vi "TCP Client_Get data signals.vi"(6 "error in":errorcluster, 7 "timeout ms":i32, 8 "hostname":string, 9 "Port":i32) -> (0 "error out":errorcluster, 1 "Array2D":sgl[][](array[numeric]), 2 "Array":sgl[](array[numeric]), 3 "Signals_names":string[](array[string]))   [LabVIEW 2022 SP3]
panel:
  out "R_message 1":string
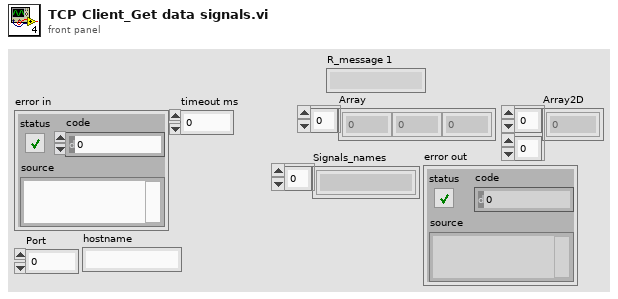
[diagram p1: front panel]
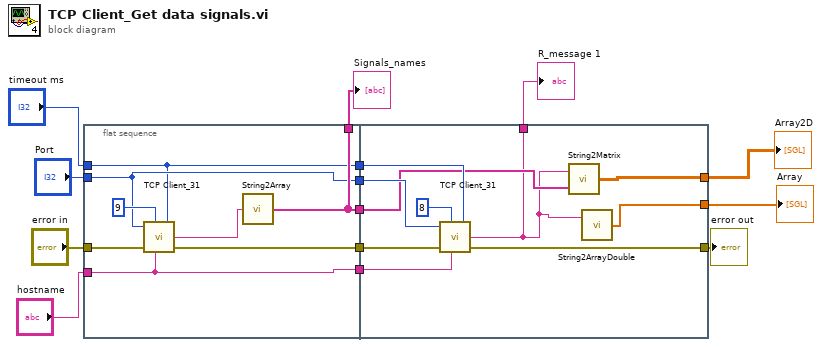
[diagram p0: block diagram]
diagram:
  n1 = flat-sequence {
    tunnel: [w18] -> w14
    tunnel: "error in" -> [w20]
    tunnel: [w19] -> w13
    tunnel: [w18] -> w5
    tunnel: "Port" -> [w17]
    tunnel: [w17] -> w10
    tunnel: "hostname" -> [w16]
    tunnel: [w16] -> w8
    tunnel: "timeout ms" -> [w15]
    tunnel: [w15] -> w6
    tunnel: w14 -> [w25]
    tunnel: w13 -> [w32]
    tunnel: [w31] -> w4
    tunnel: w10 -> [w29]
    tunnel: w8 -> [w28]
    tunnel: w6 -> [w27]
    tunnel: [w26] -> w1
    tunnel: [w24] -> w3
    tunnel: [w23] -> w2
    frame #0 {
      n2 = call "TCP Client_31.vi"("remote port or service name"=w17, "Cmd"=i8 9, "error in (no error)"=w20, "Address"=w16, "timeout ms"=w15) -> ("R_message 1"=w22:string, "error out"=w19:errorcluster)  [unwired: 1 in]
      n3 = call "String2Array.vi"("R_message 1"=w22) -> ("Array 2"=w18:string[])
    }
    frame #1 {
      n4 = call "TCP Client_31.vi"("remote port or service name"=w29, "Cmd"=u32 8 ("Cols"), "error in (no error)"=w32, "Address"=w28, "timeout ms"=w27) -> ("R_message 1"=w24:string, "error out"=w31:errorcluster)  [unwired: 1 in]
      n5 = call "String2Matrix.vi"("Header"=w25, "R_message 1"=w24) -> ("Array 3"=w26:sgl[][])
      n6 = call "String2ArrayDouble.vi"("R_message 1"=w24) -> ("Array"=w23:sgl[])  [unwired: 1 in]
    }
  }
  "Signals_names" <- w5
  "error out" <- w4
  "R_message 1" <- w3
  "Array" <- w2
  "Array2D" <- w1
